vi "Trigger Pulse.vi"() -> ()   [LabVIEW 2016]
uses:
  <vilib>/DAQmx/write.llb/DAQmx Write (Digital Bool 1Line 1Point).vi
  <vilib>/DAQmx/create/channels.llb/DAQmx Create Channel (DO-Digital Output).vi
  <vilib>/DAQmx/miscellaneous.llb/DAQmx Fill In Error Info.vi
panel:
  in  "Line":string="/port1/line1"
  in  "DAQmx Device Name":tag
  in  "Duration":dbl=0.01 format="%#_6ps"
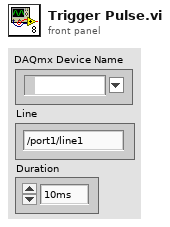
[diagram p1: front panel]
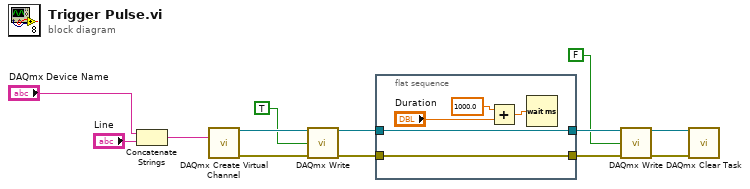
[diagram p0: block diagram]
diagram:
  n1 = Concatenate Strings("DAQmx Device Name", "Line") -> (w2:string)
  n2 = call-poly <vilib>:"DAQmx Create Virtual Channel.vi"("lines"=w2) -> ("task out"=w13:refnum<k21>, "error out"=w12:errorcluster)  [unwired: 13 in]
  n3 = call-poly <vilib>:"DAQmx Write.vi"("task/channels in"=w13, "data"=TRUE, "error in"=w12) -> ("task out"=w9:refnum<k21>, "error out"=w10:errorcluster)  [unwired: 10 in, 1 out]
  n4 = flat-sequence {
    tunnel: w10 -> [w16]
    tunnel: w9 -> [w17]
    tunnel: [w17] -> w7
    tunnel: [w16] -> w8
    frame #0 {
      n5 = Add(x=1000.0, y="Duration") -> (x+y=w15:dbl)
      n6 = Wait (ms)(milliseconds to wait=w15) -> ()  [unwired: 1 out]
    }
  }
  n7 = call-poly <vilib>:"DAQmx Write.vi"("task/channels in"=w7, "data"=FALSE, "error in"=w8) -> ("task out"=w4:refnum<k21>, "error out"=w5:errorcluster)  [unwired: 10 in, 1 out]
  n8 = call <vilib>:"DAQmx Clear Task.vi"("task in"=w4, "error in"=w5) -> ()  [unwired: 13 in, 1 out]
